vi "Calculate Scalar-Mixer Calibration Coefficients.vi"(7 "Channel (1)":i32=1, 8 "error in (no error)":errorcluster, 11 "VISA resource name":refnum<visa-resource-name>) -> (0 "error out":errorcluster, 3 "VISA resource name out":refnum<visa-resource-name>)   [LabVIEW 2018, in "Agilent ENA Series.lvlib"]
doc: "Calculates the error coefficient, from the measured calibration data, for the calibration type selected with Configure Scalar Mixer Calibration VI.\n\n<b>Notes:</b>\nAfter the error coefficient is calculated, the measured data and the calibration type setting are cleared.\n\nThis VI is not supported by the E5063A or E5080A."
uses:
  Agilent ENA Series.lvlib
panel:
  # "Note:\nThis VI is not supported by the E5063A or E5080A."
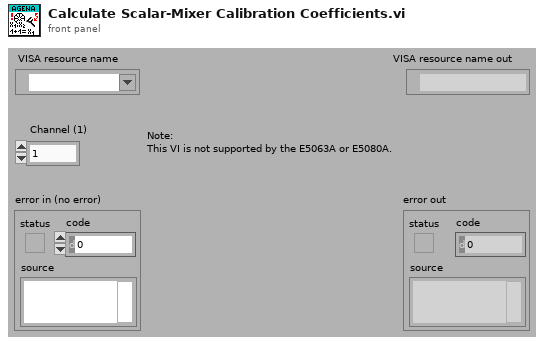
[diagram p1: front panel]
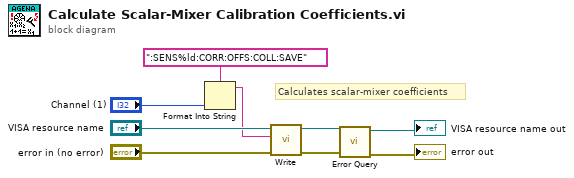
[diagram p0: block diagram]
diagram:
  # "Calculates scalar-mixer coefficients"
  n1 = Format Into String(format string=":SENS%ld:CORR:OFFS:COLL:SAVE", "Channel (1)") -> (resulting string=w5:string)  [unwired: 2 in, 1 out]
  n2 = call "Write.vi"("error in (no error)"="error in (no error)", "String ()"=w5, "VISA resource name"="VISA resource name") -> ("error out"=w3:errorcluster, "VISA resource name out"=w4:refnum<visa-resource-name>)  [unwired: 6 in, 1 out]
  n3 = call "Error Query.vi"("error in (no error)"=w3, "VISA resource name"=w4) -> ("error out"=→"error out":errorcluster, "VISA resource name out"=→"VISA resource name out":refnum<visa-resource-name>)  [unwired: 6 in, 2 out]
